vi "ParseTest.vi"() -> ()   [LabVIEW 2016]
uses:
  ClusterTypedef.ctl
  <userlib>/LevyLab/Krohn Hite 7008/SMOs/KH7008/typedefs/KH_control_array.ctl
  <userlib>/LevyLab/Krohn Hite 7008/SMOs/KH7008/typedefs/KH_control.ctl
  <userlib>/LevyLab/Krohn Hite 7008/SMOs/KH7008/typedefs/Channel-Enum.ctl
  <userlib>/LevyLab/Krohn Hite 7008/SMOs/KH7008/typedefs/Gain-Enum.ctl
  <userlib>/LevyLab/Krohn Hite 7008/SMOs/KH7008/typedefs/Shunt-Enum.ctl
  <userlib>/LevyLab/Krohn Hite 7008/SMOs/KH7008/typedefs/Input Configuration-Enum.ctl
  <userlib>/LevyLab/Krohn Hite 7008/SMOs/KH7008/KH7008.lvclass
panel:
  out "parsed output":T1={"sample"="no", "canvas"="maybe", "date"="", "user"="", "project"="", "path"=path "", "device"="", "Channel Setting"=[], "Radio Buttons"=enum."all differential", "Lockin Ch"=[], "KH Ch"=[], "Gain"=[], "Configuration"=[], "Shunt Resistor"=[], "Electrode"=[], "Label"=[]}
  out "data 2":variant
  out "items":cluster{"key":variant, "value":variant}[](array[cluster])
  in  "YAML in":string
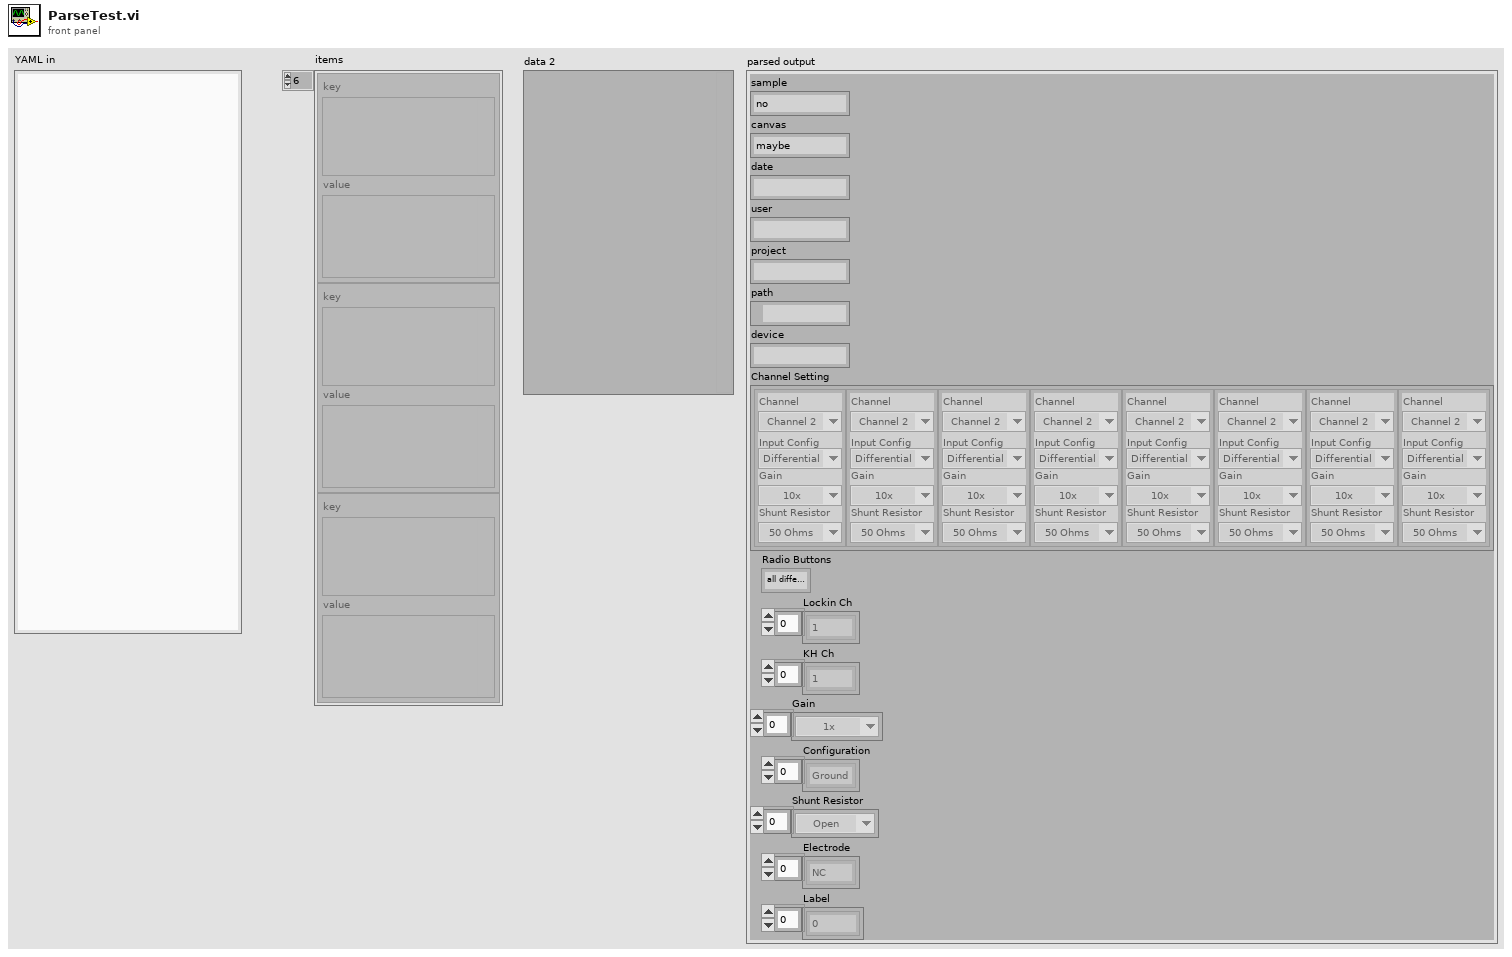
[diagram p1: front panel]
types:
  T1 = typedef "ClusterTypedef.ctl" = cluster{"sample":string, "canvas":string, "date":string, "user":string, "project":string, "path":path, "device":string, "Channel Setting":T2, "Radio Buttons":enum32{"No Selection", "all ground", "all differential"}, "Lockin Ch":enum16{"1", "2", "3", "4", "5", "6", "7", "8"}[], "KH Ch":enum16{"1", "2", "3", "4", "5", "6", "7", "8"}[], "Gain":T5[], "Configuration":enum16{"Ground", "Current", "Voltage", "Gate"}[], "Shunt Resistor":T6[], "Electrode":enum16{"NC", "26", "27", "28", "1", "2", "3", "4", "5", "6", "7", "8", "9", "10", "11", "12", "13", "14", "15", "16", "17", "18", "19", "20", "21", "22", "23", "24", "25"}[], "Label":u16[]}
  T2 = typedef "KH7008.lvclass/KH_control_array.ctl" = T3[]
  T3 = typedef "KH7008.lvclass/KH_control.ctl" = cluster{"Channel":T4, "Gain":T5, "Shunt Resistor":T6, "Input Config":T7}
  T4 = typedef "KH7008.lvclass/Channel-Enum.ctl" = enum16{"Channel 1", "Channel 2", "Channel 3", "Channel 4", "Channel 5", "Channel 6", "Channel 7", "Channel 8"}
  T5 = typedef "KH7008.lvclass/Gain-Enum.ctl" = enum16{"1x", "10x", "100x", "1000x"}
  T6 = typedef "KH7008.lvclass/Shunt-Enum.ctl" = enum16{"Open", "50 Ohms", "500 Ohms", "5k Ohms", "50k Ohms"}
  T7 = typedef "KH7008.lvclass/Input Configuration-Enum.ctl" = enum16{"Ground", "SE+ (-gnd)", "SE- (+gnd)", "Differential"}
  T8 = typedef "Dictionary Object RefNum__ogtk.ctl" = refnum<k1>
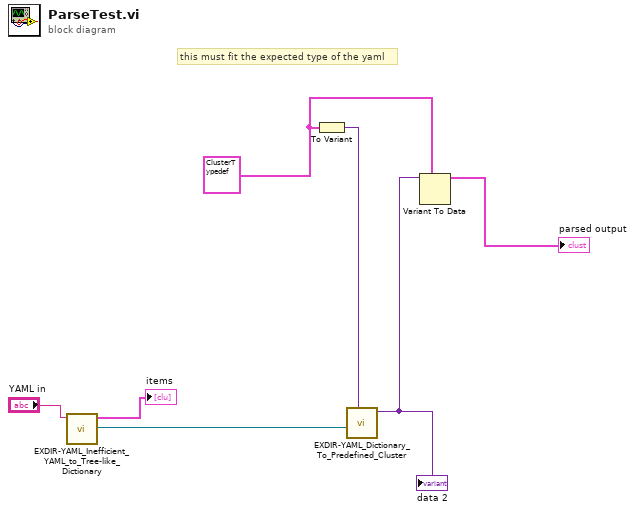
[diagram p0: block diagram]
diagram:
  w3 = T1 {"sample"="no", "canvas"="maybe", "date"="", "user"="", "project"="", "path"=path "", "device"="", "Channel Setting"=[], "Radio Buttons"=enum."all differential", "Lockin Ch"=[], "KH Ch"=[], "Gain"=[], "Configuration"=[], "Shunt Resistor"=[], "Electrode"=[], "Label"=[]} ("cluster type")
  # "this must fit the expected type of the yaml"
  n1 = call "EXDIR-YAML_Inefficient_YAML_to_Tree-like_Dictionary.vi"("YAML in"="YAML in") -> ("dictionary out"=w7:T8, "items"=→"items":cluster{"key":variant, "value":variant}[])  [unwired: 8 in]
  n2 = To Variant(anything=w3) -> (Variant=w5:variant)
  n3 = call "EXDIR-YAML_Dictionary_To_Predefined_Cluster.vi"("Cluster Type"=w5, "dictionary"=w7) -> ("VCluster out"=w4:variant)  [unwired: 8 in, 1 out]
  "data 2" <- w4
  n4 = Variant To Data(type=w3, Variant=w4) -> (data=→"parsed output":T1)  [unwired: 1 in, 1 out]
